vi "Test - JSON Minify.vi"(8 "error in":errorcluster) -> (0 "error out":errorcluster)   [LabVIEW 2020]
uses:
  <vilib>/addons/_JKI Toolkits/Caraya/classes/Assert/Assert Equal Value and Type_Variant.vi
  <vilib>/addons/_JKI Toolkits/Caraya/classes/Test/Test.lvclass
  <vilib>/addons/_JKI Toolkits/Caraya/classes/Assert/Assert.lvclass
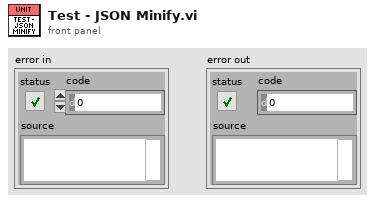
[diagram p1: front panel]
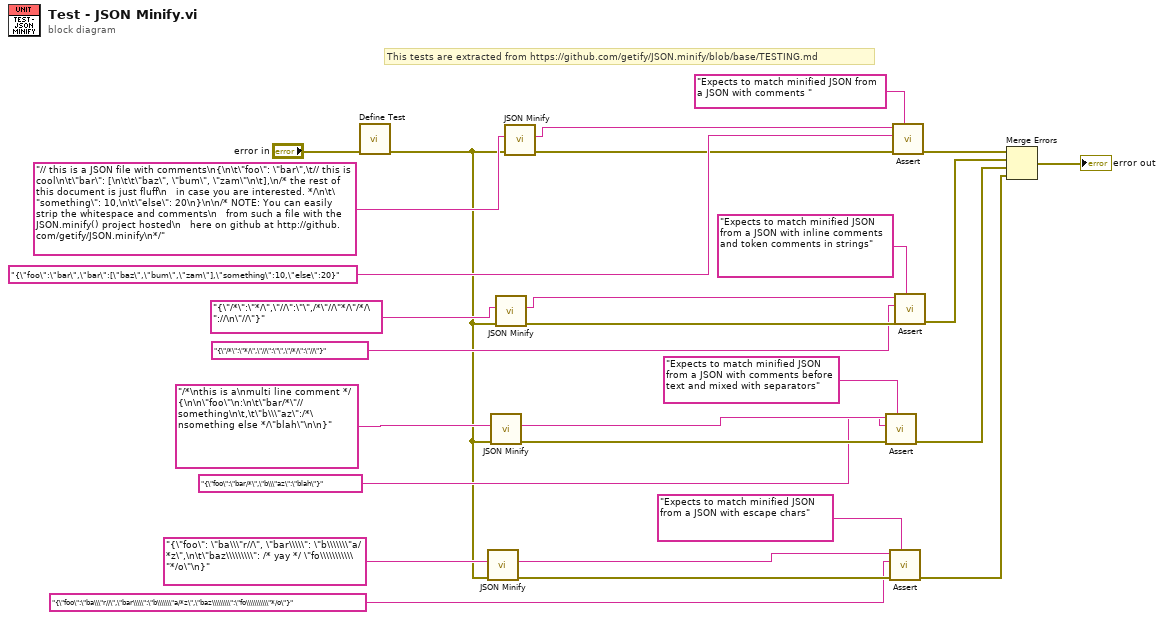
[diagram p0: block diagram]
diagram:
  # "This tests are extracted from https://github.com/getify/JSON.minify/blob/base/TESTING.md"
  n1 = call <vilib>:"Define Test.vi"("error in (no error)"="error in") -> ("error out"=w6:errorcluster)  [unwired: 10 in]
  n2 = call "JSON Minify.vi"("error in"=w6, "JSON String"="{\"foo\": \"ba\\\"r//\", \"bar\\\\\": \"b\\\\\\\"a/*z\",\n\t\"baz\\\\\\\\\": /* yay */ \"fo\\\\\\\\\\\"*/o\"\n}") -> ("error out"=w5:errorcluster, "JSON Minified"=w4:string)  [unwired: 8 in]
  n3 = call "JSON Minify.vi"("error in"=w6, "JSON String"="/*\nthis is a\nmulti line comment */{\n\n\"foo\"\n:\n\t\"bar/*\"// something\n\t,\t\"b\\\"az\":/*\nsomething else */\"blah\"\n\n}") -> ("error out"=w12:errorcluster, "JSON Minified"=w11:string)  [unwired: 8 in]
  n4 = call "JSON Minify.vi"("error in"=w6, "JSON String"="{\"/*\":\"*/\",\"//\":\"\",/*\"//\"*/\"/*/\"://\n\"//\"}") -> ("error out"=w18:errorcluster, "JSON Minified"=w19:string)  [unwired: 8 in]
  n5 = call "JSON Minify.vi"("JSON String"="// this is a JSON file with comments\n{\n\t\"foo\": \"bar\",\t// this is cool\n\t\"bar\": [\n\t\t\"baz\", \"bum\", \"zam\"\n\t],\n/* the rest of this document is just fluff\n   in case you are interested. */\n\t\"something\": 10,\n\t\"else\": 20\n}\n\n/* NOTE: You can easily strip the whitespace and comments\n   from such a file with the JSON.minify() project hosted\n   here on github at http://github.com/getify/JSON.minify\n*/") -> ("JSON Minified"=w21:string)  [unwired: 9 in, 1 out]
  n6 = call-poly <vilib>:"Assert.vi"("Label"="Expects to match minified JSON from a JSON with comments before text and mixed with separators" ("Label (VI Title)"), "error in (no error)"=w12, "Y"="{\"foo\":\"bar/*\",\"b\\\"az\":\"blah\"}", "X"=w11) -> ("error out"=w8:errorcluster)  [unwired: 7 in]
  n7 = call-poly <vilib>:"Assert.vi"("Label"="Expects to match minified JSON from a JSON with escape chars" ("Label (VI Title)"), "error in (no error)"=w5, "Y"="{\"foo\":\"ba\\\"r//\",\"bar\\\\\":\"b\\\\\\\"a/*z\",\"baz\\\\\\\\\":\"fo\\\\\\\\\\\"*/o\"}", "X"=w4) -> ("error out"=w2:errorcluster)  [unwired: 7 in]
  n8 = call-poly <vilib>:"Assert.vi"("Label"="Expects to match minified JSON from a JSON with comments " ("Label (VI Title)"), "error in (no error)"=w6, "Y"="{\"foo\":\"bar\",\"bar\":[\"baz\",\"bum\",\"zam\"],\"something\":10,\"else\":20}" ("JSON Minified"), "X"=w21) -> ("error out"=w25:errorcluster)  [unwired: 7 in]
  n9 = call-poly <vilib>:"Assert.vi"("Label"="Expects to match minified JSON from a JSON with inline comments and token comments in strings" ("Label (VI Title)"), "error in (no error)"=w18, "Y"="{\"/*\":\"*/\",\"//\":\"\",\"/*/\":\"//\"}", "X"=w19) -> ("error out"=w17:errorcluster)  [unwired: 7 in]
  n10 = Merge Errors(w25, w17, w8, w2) -> (→"error out":errorcluster)
